vi "Host3.vi"() -> ()   [LabVIEW 2025]
uses:
  <vilib>/numeric/Random Number (Range) U64.vi
  <vilib>/Analysis/baseanly.llb/Real Dot Product.vi
  <vilib>/Analysis/baseanly.llb/Real A x B.vi
  <vilib>/numeric/sub_Random U32.vi
  <vilib>/Analysis/Matrix/Numeric/Conversions/Matrix To Array - RM.vi
  <vilib>/FPGAPlugInAG/cRIO-9033/niLvFpga_Open_cRIO-9033.vi
  <vilib>/rvi/interface/common/dynamic/niFpgaDynamicAddResources.vi
  <vilib>/FPGAPlugInAG/Dynamic/niLvFpga_Reset_Dynamic.vi
  <vilib>/Utility/error.llb/Error Cluster From Error Code.vi
  <vilib>/rvi/errors/niLvFpgaAdjustHostInterfaceError.vi
  <vilib>/FPGAPlugInAG/Dynamic/niLvFpga_Run_Dynamic.vi
  <vilib>/FPGAPlugInAG/Dynamic/niLvFpga_Close_Dynamic.vi
  <vilib>/rvi/interface/nirviOpenFPGA/nirviOpenFPGA.xnode
  FPGA Bitfiles/dotplot9033_FPGATarget_Target3_Ds7gJeQCrVA.lvbitx
  Target3.vi
  <vilib>/rvi/interface/nirviMethod/nirviMethod.xnode
  <vilib>/rvi/interface/nirviCloseFPGA/nirviCloseFPGA.xnode
  <vilib>/rvi/errors/niLvFpgaMergeErrorWithErrorCode.vi
  <vilib>/Analysis/NI_AALBase.lvlib
  <vilib>/Analysis/Matrix/NI_Matrix.lvlib
  <vilib>/FPGAPlugInAG/Dynamic/niLvFpga_ReadFifo_Dynamic.vi
  <vilib>/FPGAPlugInAG/Dynamic/niLvFpga_WriteFifo_Dynamic.vi
panel:
  out "FIFO C Output":fxp<+/-,32,16>[](array[numeric])
  out "FIFO A Input":fxp<+/-,32,16>[](array[numeric])
  out "FIFO B Input":fxp<+/-,32,16>[](array[numeric])
  out "X * Y":fxp<+/-,64,32>
  out "elements in B":i32
  out "elements in A":i32
  out "sum of error":dbl
  out "C - FPGA code":fxp<+/-,32,16>[][](array[numeric])
  out "elements in C":i32
  out "C - Real":dbl[][](array[numeric])
  out "B":fxp<+/-,32,16>[][](array[numeric])
  out "A":fxp<+/-,32,16>[][](array[numeric])
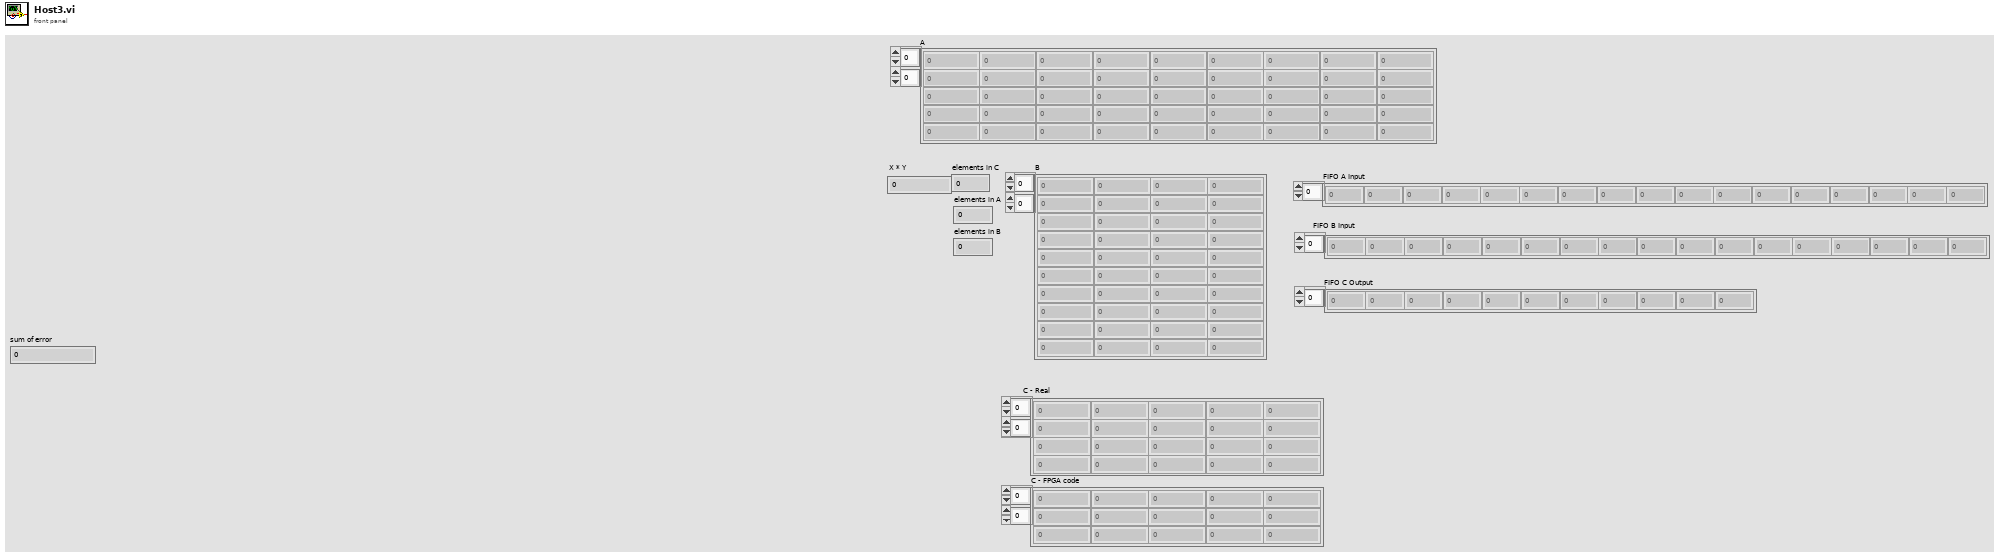
[diagram p1: front panel]
types:
  T1 = typedef "NI_Matrix.lvlib/RealMatrix.ctl" = dbl[][]
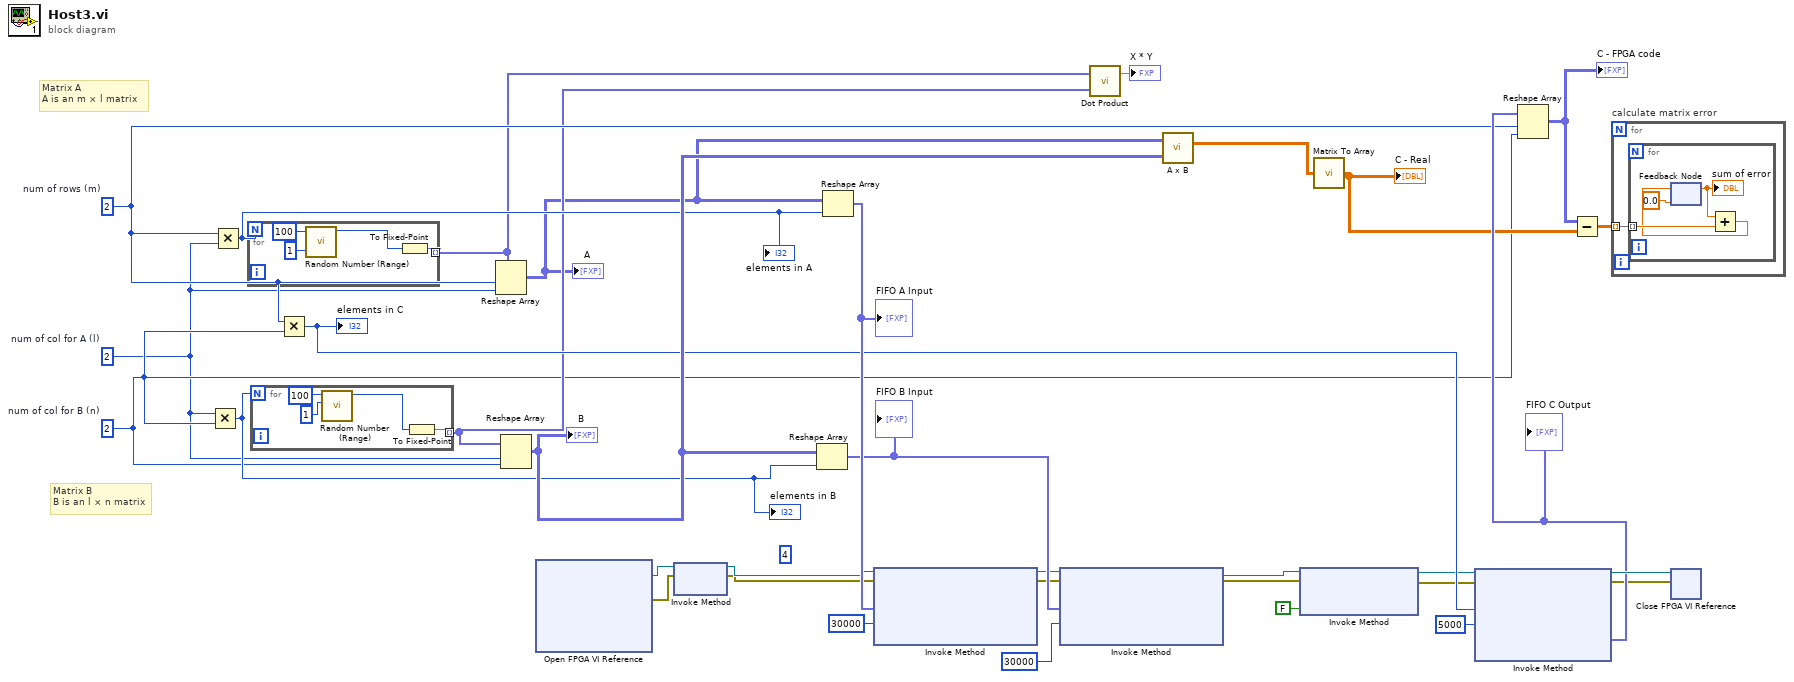
[diagram p0: block diagram]
diagram:
  (unwired) 4
  w17 = 2  # num of col for B (n)
  w16 = 2  # num of col for A (l)
  w26 = 2  # num of rows (m)
  # "Matrix B\nB is an l × n matrix"
  # "Matrix A\nA is an m × l matrix"
  n1 = Multiply(x=w16, y=w17) -> (x*y=w23:i32)
  "elements in B" <- w23
  n2 = Multiply(x=w26, y=w16) -> (x*y=w31:i32)
  "elements in A" <- w31
  n3 = for {
    N: w31 -> [_]
    tunnel: [w38] -> w22 mode=indexing
    n4 = call-poly <vilib>:"Random Number (Range).vi"("lower bound (0)"=u64 1, "upper bound (100)"=u64 100) -> ("number"=w37:u64)  [unwired: 9 in]
    n5 = To Fixed-Point(number=w37) -> (fixed-point=w38:fxp<+,64,64>)  [unwired: 1 in]
  }
  n6 = for {
    N: w23 -> [_]
    tunnel: [w42] -> w21 mode=indexing
    n7 = call-poly <vilib>:"Random Number (Range).vi"("lower bound (0)"=u64 1, "upper bound (100)"=u64 100) -> ("number"=w39:u64)  [unwired: 9 in]
    n8 = To Fixed-Point(number=w39) -> (fixed-point=w42:fxp<+,64,64>)  [unwired: 1 in]
  }
  n9 = Multiply(x=w26, y=w17) -> (x*y=w24:i32)
  "elements in C" <- w24
  n10 = Reshape Array(w22, w26, w16) -> (w18:fxp<+,64,64>[][])
  "A" <- w18
  n11 = Reshape Array(w21, w16, w17) -> (w33:fxp<+,64,64>[][])
  "B" <- w33
  n12 = xnode "Open FPGA VI Reference"() -> ("FPGA VI Reference Out"=w14:refnum<k20>, "error out"=w11:errorcluster)  [unwired: 2 in]
  n13 = xnode "Invoke Method"("FPGA VI Reference In"=w14, "error in"=w11) -> ("FPGA VI Reference Out"=w13:refnum<k20>, "error out"=w12:errorcluster)
  n14 = Reshape Array(w33, w23) -> (w15:fxp<+,64,64>[])
  "FIFO B Input" <- w15
  n15 = Reshape Array(w18, w31) -> (w30:fxp<+,64,64>[])
  "FIFO A Input" <- w30
  n16 = xnode "Invoke Method"("FPGA VI Reference In"=w13, "error in"=w12, "Data"=w30, "Timeout (ms)"=30000) -> ("FPGA VI Reference Out"=w4:refnum<k20>, "error out"=w3:errorcluster)  [unwired: 1 out]
  n17 = xnode "Invoke Method"("FPGA VI Reference In"=w4, "error in"=w3, "Data"=w15, "Timeout (ms)"=30000) -> ("FPGA VI Reference Out"=w7:refnum<k20>, "error out"=w6:errorcluster)  [unwired: 1 out]
  n18 = call-poly <vilib>:"Dot Product.vi"("Y Vector"=w21, "X Vector"=w22) -> ("X * Y"=→"X * Y":dbl)  [unwired: 1 out]
  n19 = call-poly <vilib>:"A x B.vi"("B"=w33, "A"=w18) -> ("A x B"=w32:T1)  [unwired: 1 out]
  n20 = xnode "Invoke Method"("FPGA VI Reference In"=w7, "error in"=w6, "Wait Until Done (F)"=FALSE) -> ("FPGA VI Reference Out"=w9:refnum<k20>, "error out"=w8:errorcluster)
  n21 = call-poly <vilib>:"Matrix To Array.vi"("Real Matrix"=w32) -> ("Real 2D Array"=w25:dbl[][])
  "C - Real" <- w25
  n22 = xnode "Invoke Method"("FPGA VI Reference In"=w9, "error in"=w8, "Number of Elements"=w24, "Timeout (ms)"=5000) -> ("FPGA VI Reference Out"=w34:refnum<k20>, "error out"=w19:errorcluster, "Data"=w27:fxp<+/-,32,16>[])  [unwired: 1 out]
  "FIFO C Output" <- w27
  n23 = Reshape Array(w27, w26, w17) -> (w29:fxp<+/-,32,16>[][])
  "C - FPGA code" <- w29
  n24 = Subtract(x=w29, y=w25) -> (x-y=w28:dbl[][])
  n25 = for "calculate matrix error" {
    tunnel: w28 -> [w43] mode=indexing
    n26 = for {
      tunnel: w43 -> [w47] mode=indexing
      n27 = feedback #1(0.0) -> (w45:dbl)
      "sum of error" <- w45
      n28 = Add(x=w45, y=w47) -> (x+y=w46:dbl)
      n29 = feedback-in #1(w46) -> ()
    }
  }
  n30 = xnode "Close FPGA VI Reference"("FPGA VI Reference In"=w34, "error in"=w19) -> ()  [unwired: 1 out]
